vi "Check if Rock.vi"(5 "Rock Positions":cluster{i32, i32}[](array[cluster]), 6 "Grid Size":cluster{"number of columns":i32, "matrix":i32}, 7 "Current Positions":set{cluster{i32, i32}}(c389), 10 "Knowns Rocks":set{cluster{i32, i32}}(c389), 11 "Known Good Positions In":set{cluster{i32, i32}}(c389)) -> (2 "Known Rocks Out":set{cluster{i32, i32}}(c389), 3 "Known Good Positions Out":set{cluster{i32, i32}}(c389))   [LabVIEW 2021]
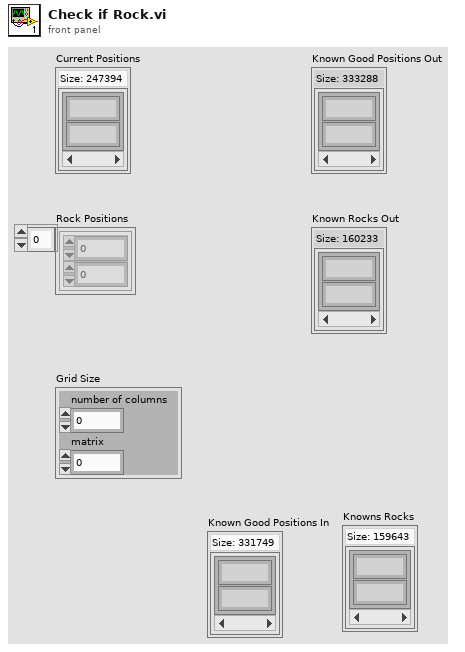
[diagram p1: front panel]
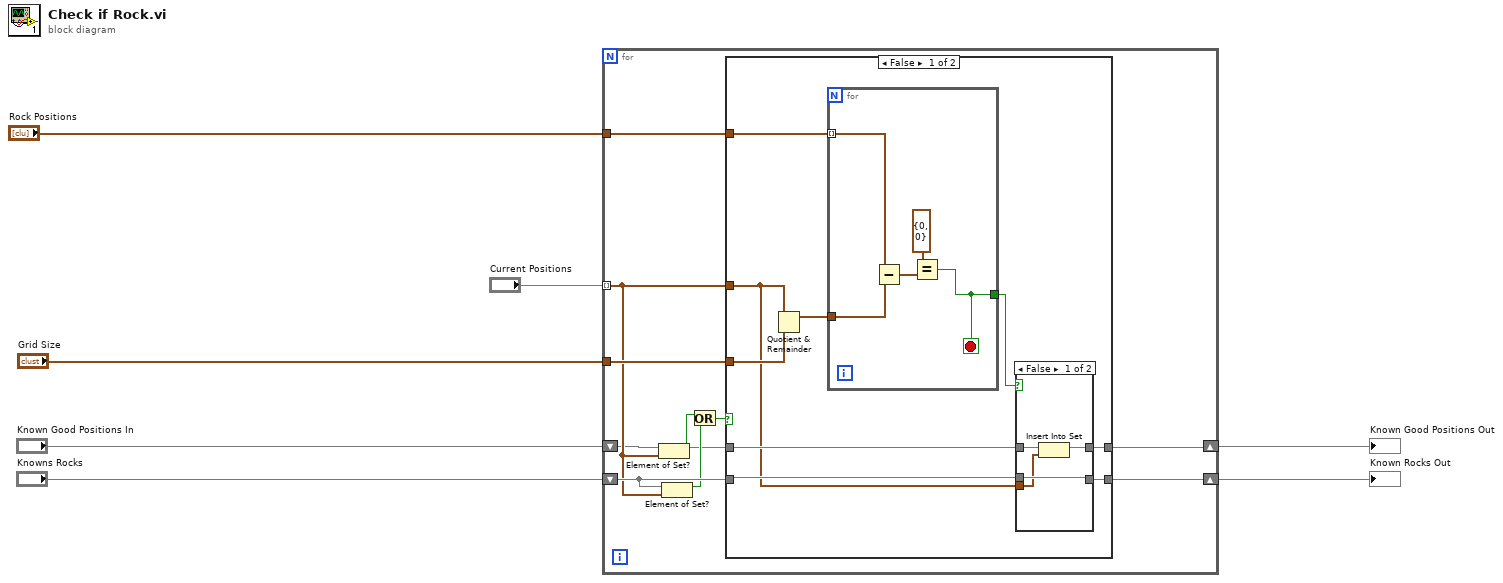
[diagram p0: block diagram]
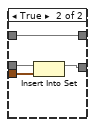
[diagram p2: hidden frame]
diagram:
  n1 = for {
    tunnel: "Current Positions" -> [w13] mode=indexing
    tunnel: "Rock Positions" -> [w17]
    tunnel: "Grid Size" -> [w16]
    shift-right: [w14] -> w5
    shift-left: "Knowns Rocks" -> [w15]
    shift-right: [w9] -> w7
    shift-left: "Known Good Positions In" -> [w8]
    n2 = Element of Set?(10:w13, 11:w8) -> (3:w12:bool)
    n3 = Element of Set?(10:w13, 11:w15) -> (3:w11:bool)
    n4 = Or(x=w12, y=w11) -> (x .or. y?=w10:bool)
    n5 = case shown="False" w10 {
      tunnel: w17 -> [w26 _]
      tunnel: w16 -> [w25 _]
      tunnel: w13 -> [w18 _]
      tunnel: w15 -> [w23 w41]
      tunnel: [w22 w41] -> w14
      tunnel: [w19 w40] -> w9
      tunnel: w8 -> [w20 w40]
      frame False {
        n6 = Quotient & Remainder(x=w18, y=w25) -> (x-y*floor(x/y)=w24:cluster{i32, i32})  [unwired: 1 out]
        n7 = for {
          tunnel: w26 -> [w37] mode=indexing
          tunnel: [w39] -> w21
          tunnel: w24 -> [w38]
          stop <- w39 stop-if-true
          n8 = Subtract(x=w37, y=w38) -> (x-y=w36:cluster{i32, i32})
          n9 = Equal?(x=cluster{i32, i32} {0, 0}, y=w36) -> (x = y?=w39:bool)
        }
        n10 = case shown="False" w21 {
          tunnel: w23 -> [w30 w34]
          tunnel: [w30 w33] -> w22
          tunnel: w20 -> [w29 w32]
          tunnel: [w28 w32] -> w19
          tunnel: w18 -> [w27 w31]
          frame False {
            n11 = Insert Into Set(10:w27, 11:w29) -> (3:w28:set{cluster{i32, i32}})  [unwired: 1 out]
          }
          frame True {
            n12 = Insert Into Set(10:w31, 11:w34) -> (3:w33:set{cluster{i32, i32}})  [unwired: 1 out]
          }
        }
      }
      frame True {
      }
    }
  }
  "Known Good Positions Out" <- w7
  "Known Rocks Out" <- w5
